vi "aptMotorControl_AutoInput.vi"() -> ()   [LabVIEW 2013]
panel:
  out "Z Location":sgl
  in  "Z Input":dbl
  out "pfPosition 3":sgl
  out "pfPosition 2":sgl
  in  "Serial 3":i32=90848556
  in  "MG17Motor 3":refnum<k7>(container)
  in  "Serial 2":i32=90848555
  in  "MG17Motor 2":refnum<k7>(container)
  in  "MG17Motor":refnum<k7>(container)
  in  "stop":bool
  in  "Serial":i32=90848557
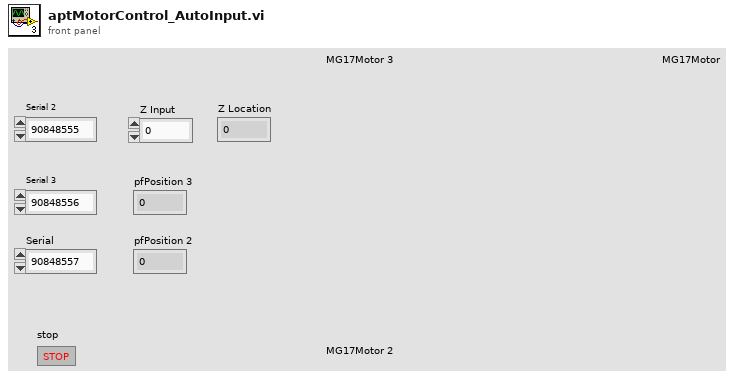
[diagram p1: front panel]
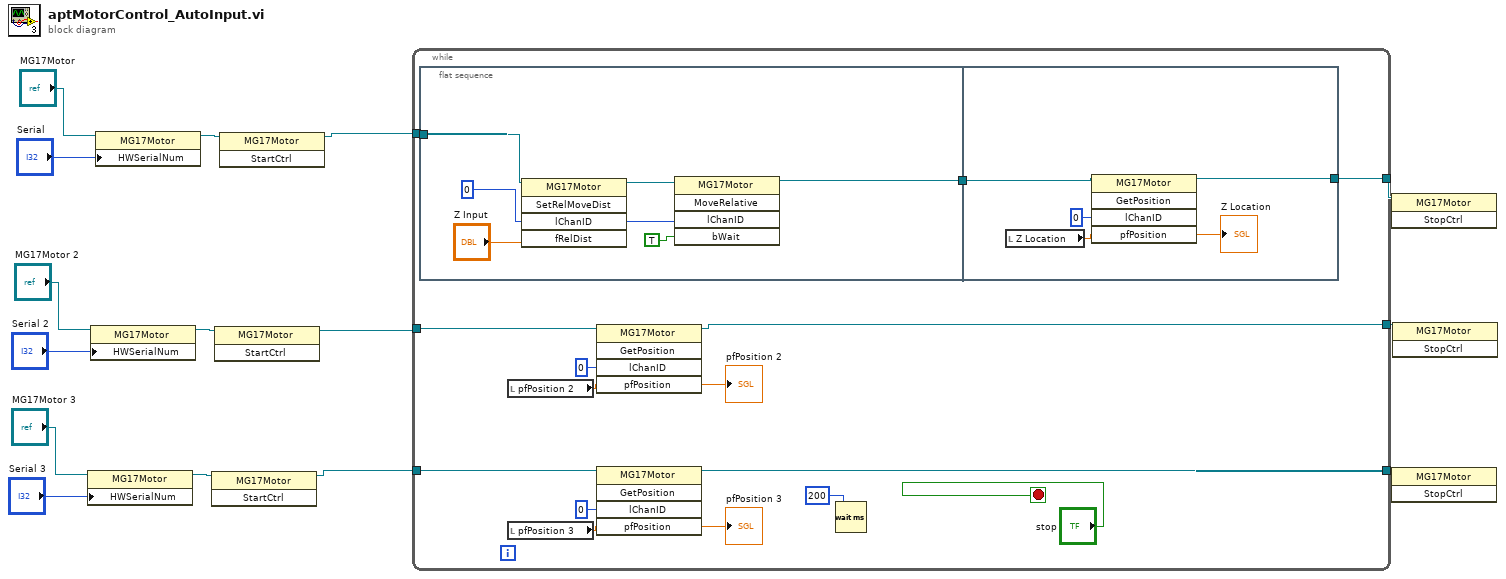
[diagram p0: block diagram]
diagram:
  n1 = property class="MG17Motor"(reference="MG17Motor 3", "HWSerialNum"="Serial 3") -> (reference out=w6:refnum<k7>)  [unwired: 1 in, 1 out]
  n2 = property class="MG17Motor"(reference="MG17Motor 2", "HWSerialNum"="Serial 2") -> (reference out=w9:refnum<k7>)  [unwired: 1 in, 1 out]
  n3 = property class="MG17Motor"(reference="MG17Motor", "HWSerialNum"="Serial") -> (reference out=w12:refnum<k7>)  [unwired: 1 in, 1 out]
  n4 = invoke class="MG17Motor" method="StartCtrl"(reference=w6) -> (reference out=w3:refnum<k7>)  [unwired: 2 in, 2 out]
  n5 = invoke class="MG17Motor" method="StartCtrl"(reference=w9) -> (reference out=w5:refnum<k7>)  [unwired: 2 in, 2 out]
  n6 = invoke class="MG17Motor" method="StartCtrl"(reference=w12) -> (reference out=w13:refnum<k7>)  [unwired: 2 in, 2 out]
  n7 = while {
    tunnel: w13 -> [w18]
    tunnel: w5 -> [w25]
    tunnel: [w24] -> w4
    tunnel: w3 -> [w20]
    tunnel: [w19] -> w2
    tunnel: [w17] -> w1
    stop <- "stop" stop-if-true
    n8 = flat-sequence {
      tunnel: w18 -> [w33]
      tunnel: [w31] -> w16
      tunnel: [w39] -> w17
      tunnel: w16 -> [w38]
      frame #0 {
        n9 = invoke class="MG17Motor" method="SetRelMoveDist"(reference=w33, "lChanID"=0, "fRelDist"="Z Input") -> (reference out=w37:refnum<k7>, "lChanID"=w36:i32)  [unwired: 2 in, 3 out]
        n10 = invoke class="MG17Motor" method="MoveRelative"(reference=w37, "lChanID"=w36, "bWait"=TRUE) -> (reference out=w31:refnum<k7>)  [unwired: 2 in, 4 out]
      }
      frame #1 {
        n11 = local read "Z Location"() -> (w42:sgl)
        n12 = invoke class="MG17Motor" method="GetPosition"(reference=w38, "lChanID"=0, "pfPosition"=w42) -> (reference out=w39:refnum<k7>, "pfPosition"=→"Z Location":sgl)  [unwired: 2 in, 3 out]
      }
    }
    n13 = local read "pfPosition 2"() -> (w28:sgl)
    n14 = local read "pfPosition 3"() -> (w21:sgl)
    n15 = invoke class="MG17Motor" method="GetPosition"(reference=w25, "lChanID"=0, "pfPosition"=w28) -> (reference out=w24:refnum<k7>, "pfPosition"=→"pfPosition 2":sgl)  [unwired: 2 in, 3 out]
    n16 = invoke class="MG17Motor" method="GetPosition"(reference=w20, "lChanID"=0, "pfPosition"=w21) -> (reference out=w19:refnum<k7>, "pfPosition"=→"pfPosition 3":sgl)  [unwired: 2 in, 3 out]
    n17 = Wait (ms)(milliseconds to wait=u32 200) -> ()  [unwired: 1 out]
  }
  n18 = invoke class="MG17Motor" method="StopCtrl"(reference=w1) -> ()  [unwired: 2 in, 3 out]
  n19 = invoke class="MG17Motor" method="StopCtrl"(reference=w2) -> ()  [unwired: 2 in, 3 out]
  n20 = invoke class="MG17Motor" method="StopCtrl"(reference=w4) -> ()  [unwired: 2 in, 3 out]
